vi "题目3.vi"() -> ()   [LabVIEW 2017]
panel:
  out "波形图":dbl[][](graph)
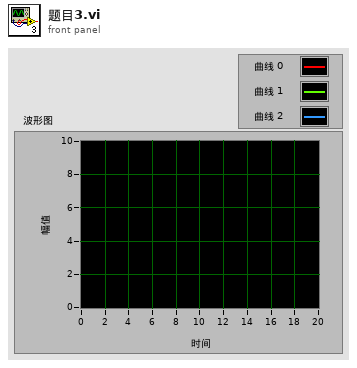
[diagram p1: front panel]
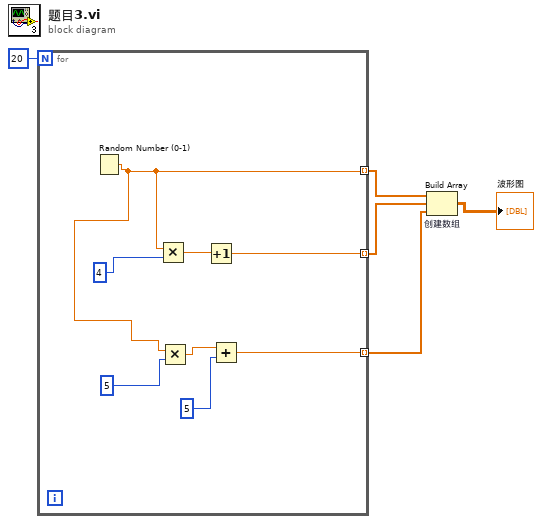
[diagram p0: block diagram]
diagram:
  n1 = for {
    N: 20 -> [_]
    tunnel: [w6] -> w5 mode=indexing
    tunnel: [w8] -> w4 mode=indexing
    tunnel: [w7] -> w3 mode=indexing
    n2 = Random Number (0-1)() -> (number: 0 to 1=w6:dbl)
    n3 = Multiply(x=w6, y=4) -> (x*y=w11:dbl)
    n4 = Multiply(x=w6, y=5) -> (x*y=w10:dbl)
    n5 = Increment(x=w11) -> (x+1=w8:dbl)
    n6 = Add(x=w10, y=5) -> (x+y=w7:dbl)
  }
  n7 = Build Array "创建数组"(w5, w4, w3) -> (→"波形图":dbl[][])
